vi "Acceleration Limiter.vi"(4 "Max Decel (NU/s); 0 for -accel":dbl, 5 "Max Accel (Native Units/s)":dbl, 6 "Current Time":dbl, 8 "Target Speed":dbl) -> (2 "Adjusted Target":dbl)   [LabVIEW 2015]
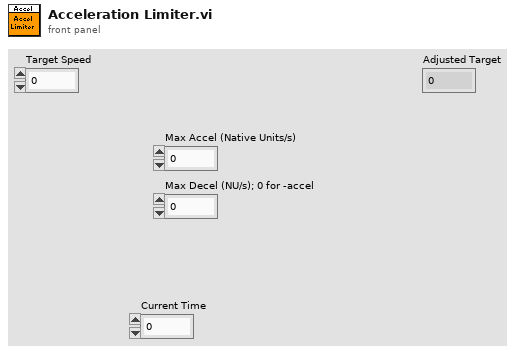
[diagram p1: front panel]
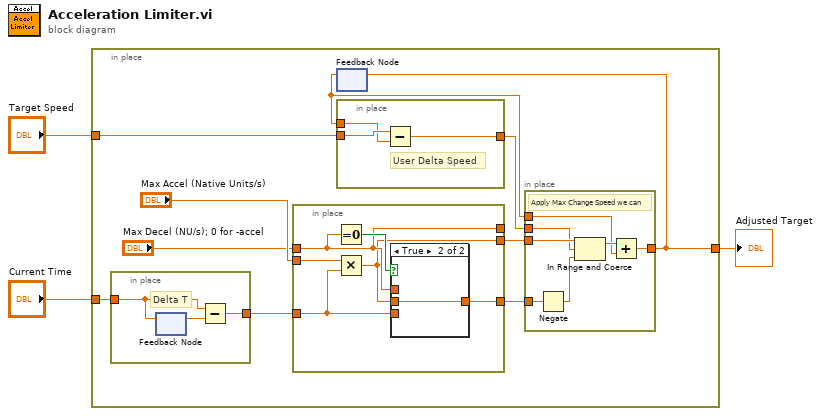
[diagram p0: block diagram]
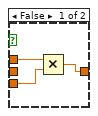
[diagram p2: hidden frame]
diagram:
  n1 = in-place {
    in-place-border: "Current Time" -> [w13]
    in-place-border: "Target Speed" -> [w9]
    in-place-border: [w8] -> w2
    n2 = in-place {
      in-place-border: w13 -> [w32]
      in-place-border: [w31] -> w12
      # "Delta T"
      n3 = feedback #1() -> (w33:dbl)  [unwired: 1 in]
      n4 = feedback-in #1(w32) -> ()
      n5 = Subtract(x=w32, y=w33) -> (x-y=w31:dbl)
    }
    n6 = in-place {
      in-place-border: "Max Accel (Native Units/s)" -> [w22]
      in-place-border: w12 -> [w26]
      in-place-border: [w21] -> w11
      in-place-border: [w23] -> _
      in-place-border: [w25] -> w5
      in-place-border: "Max Decel (NU/s); 0 for -accel" -> [w23]
      n7 = Equal To 0?(x=w23) -> (x = 0?=w24:bool)
      n8 = Multiply(x=w22, y=w26) -> (x*y=w21:dbl)
      n9 = case shown="True" w24 {
        tunnel: w23 -> [w29 _]
        tunnel: w26 -> [w28 _]
        tunnel: [w27 w30] -> w25
        tunnel: w21 -> [_ w30]
        frame False {
          n10 = Multiply(x=w29, y=w28) -> (x*y=w27:dbl)
        }
        frame True {
        }
      }
    }
    n11 = feedback #2() -> (w7:dbl)  [unwired: 1 in]
    n12 = in-place {
      in-place-border: w9 -> [w36]
      in-place-border: [w35] -> w10
      in-place-border: w7 -> [w34]
      # "User Delta Speed"
      n13 = Subtract(x=w36, y=w34) -> (x-y=w35:dbl)
    }
    n14 = in-place {
      in-place-border: w11 -> [w20]
      in-place-border: w10 -> [w19]
      in-place-border: w7 -> [w17]
      in-place-border: [w16] -> w8
      in-place-border: w5 -> [w14]
      # "Apply Max Change Speed we can"
      n15 = Negate(x=w14) -> (-x=w15:dbl)
      n16 = In Range and Coerce(upper limit=w20, x=w19, lower limit=w15) -> (coerced(x)=w18:dbl)  [unwired: 1 out]
      n17 = Add(x=w18, y=w17) -> (x+y=w16:dbl)
    }
    n18 = feedback-in #2(w8) -> ()
  }
  "Adjusted Target" <- w2
